vi "Main.vi"() -> ()   [LabVIEW 2021]
uses:
  <vilib>/gmath/NumericalOptimization/stopping criteria.ctl
  <vilib>/Platform/TimedLoop/XDataNode/timing_clust.ctl
  <vilib>/Platform/TimedLoop/XDataNode/nitl_modes.ctl
  <vilib>/Platform/TimedLoop/XDataNode/wakeup.ctl
  <vilib>/DAQmx/write.llb/DAQmx Write (Digital 1D Bool 1Chan 1Samp).vi
  <vilib>/DAQmx/write.llb/DAQmx Write (Analog 1D DBL NChan 1Samp).vi
  <vilib>/DAQmx/create/channels.llb/DAQmx Create Channel (DO-Digital Output).vi
  <vilib>/DAQmx/create/channels.llb/DAQmx Create Channel (AO-Voltage-Basic).vi
  <vilib>/DAQmx/create/channels.llb/DAQmx Create Channel (AI-Voltage-Basic).vi
  <vilib>/DAQmx/configure/timing.llb/DAQmx Timing (Sample Clock).vi
  <vilib>/DAQmx/miscellaneous.llb/DAQmx Fill In Error Info.vi
  <vilib>/platform/TimedLoop/XDataNode/XDataNode.xnode
  <vilib>/Platform/TimedLoop/XDataNode/XDNodeRunTimeDep.lvlib
  <vilib>/Analysis/NI_AALBase.lvlib
  <vilib>/Analysis/baseanly.llb/Real Dot Product.vi
  <vilib>/gmath/NI_Gmath.lvlib
panel:
  in  "RBF 5":bool=TRUE
  in  "State x 3":cluster{"Number":i32, "x_0":dbl, "x_f":dbl}={"Number"=20, "x_0"=0.0, "x_f"=500.0}
  out "XY Graph 3":cluster{dbl[], dbl[]}[](graph)=[{[0.0, 26.31578947368421, 52.63157894736842, 78.94736842105263, 105.26315789473684, 131.57894736842104, 157.89473684210526, 184.21052631578945, 210.52631578947367, 236.8421052631579, 263.1578947368421, 289.4736842105263, 315.7894736842105, 342.10526315789474, 368.4210526315789, 394.7368421052631, 421.05263157894734, 447.36842105263156, 473.6842105263158, 499.99999999999994], [-1.87, -1.8414422208867078, -1.7583590718201578, -1.6281335147614857, -1.4618588659589593, -1.2727815045556152, -1.0745713204427367, -0.879730430835235, -0.6983883150844216, -0.5376223240442685, -0.40131981493157487, -0.2904938166741144, -0.20389950050143207, -0.13878048824938563, -0.09159539506910583, -0.058620814615532306, -0.03638002877625406, -0.02189309729851222, -0.012775689731560116, -0.007229270660814157]}, {[0.0, 26.31578947368421, 52.63157894736842, 78.94736842105263, 105.26315789473684, 131.57894736842104, 157.89473684210526, 184.21052631578945, 210.52631578947367, 236.8421052631579, 263.1578947368421, 289.4736842105263, 315.7894736842105, 342.10526315789474, 368.4210526315789, 394.7368421052631, 421.05263157894734, 447.36842105263156, 473.6842105263158, 499.99999999999994], [-0.5809906464511002, -0.7664296918795039, -0.9804116917090333, -1.2161233359855126, -1.462782454638376, -1.706140698730468, -1.9296694582665639, -2.116332899482121, -2.2507021378374863, -2.3210529255377237, -2.3210529255377237, -2.2507021378374863, -2.1163328994821216, -1.9296694582665639, -1.7061406987304686, -1.4627824546383765, -1.2161233359855128, -0.9804116917090334, -0.7664296918795039, -0.5809906464511005]}, {[0.0, 26.31578947368421, 52.63157894736842, 78.94736842105263, 105.26315789473684, 131.57894736842104, 157.89473684210526, 184.21052631578945, 210.52631578947367, 236.8421052631579, 263.1578947368421, 289.4736842105263, 315.7894736842105, 342.10526315789474, 368.4210526315789, 394.7368421052631, 421.05263157894734, 447.36842105263156, 473.6842105263158, 499.99999999999994], [0.006649382639893229, 0.011750901785178288, 0.020136966499166315, 0.03346184464981654, 0.05391861023460723, 0.08424817086570154, 0.12764836352349906, 0.18754392559490007, 0.2671921736253885, 0.3691283859263683, 0.49449753869312374, 0.6423678620027834, 0.8091638187361518, 0.9883757599794155, 1.1706867314629184, 1.3445974595986148, 1.4975345697271418, 1.6173142264869897, 1.6937329518316242, 1.72]}, {[0.0, 26.31578947368421, 52.63157894736842, 78.94736842105263, 105.26315789473684, 131.57894736842104, 157.89473684210526, 184.21052631578945, 210.52631578947367, 236.8421052631579, 263.1578947368421, 289.4736842105263, 315.7894736842105, 342.10526315789474, 368.4210526315789, 394.7368421052631, 421.05263157894734, 447.36842105263156, 473.6842105263158, 499.99999999999994], [-2.444341263811207, -2.5961210109810335, -2.7186337970300247, -2.8107950060971816, -2.8707227103627284, -2.8946740324203812, -2.8765924151858018, -2.808519404722456, -2.6818982792965196, -2.489546863655624, -2.2278752017761745, -1.898828092508817, -1.5110685812474018, -1.080074186536534, -0.627049362336656, -0.17680580965529402, 0.2450312049653749, 0.6150094374794441, 0.9145275702205602, 1.1317800828880853]}]
  in  "RBF 4":cluster{"STD":dbl, "Number":i32}={"STD"=150.0, "Number"=3}
  out "RBF Output 3":dbl(slide)=-2.8000715957430593 scale=-40.0..50.0
  out "Weights 3":dbl[](array[slide])=[-1.87, -2.33, 1.72] scale=0.0..100.0
  out "100ms Finished Late?":bool
  out "100ms":i64=2
  out "1ms Finished Late?":bool
  in  "Encoder":bool
  in  "Tension Control Gains":T1(array[cluster])=[{"proportional gain (Kc)"=0.03, "integral time (Ti, min)"=0.0, "derivative time (Td, min)"=0.0}, {"proportional gain (Kc)"=0.03, "integral time (Ti, min)"=0.0, "derivative time (Td, min)"=0.0}, {"proportional gain (Kc)"=0.03, "integral time (Ti, min)"=0.0, "derivative time (Td, min)"=0.0}] {"derivative time (Td, min)" format="%.3f"; "integral time (Ti, min)" format="%.3f"; "proportional gain (Kc)" format="%.3f"}
  out "Ref Position (mm)":dbl
  out "1ms":i64=2
  in  "stop":bool
  out "10ms Finished Late?":bool
  out "10ms":i64=2
  in  "QP Stopping Criteria":T2={"function tolerance"=0.001, "parameter tolerance"=1e-05, "max iterations"=50, "max function calls"=50, "gradient tolerance"=1e-05, "max time (sec)"=0.01}
  in  "QP?":bool
  out "QP Solved":bool
  in  "Record?":bool
  in  "Trajectory":i32(knob) scale=0.0..2.0
  # "CONTROL"
  # "DEVEL"
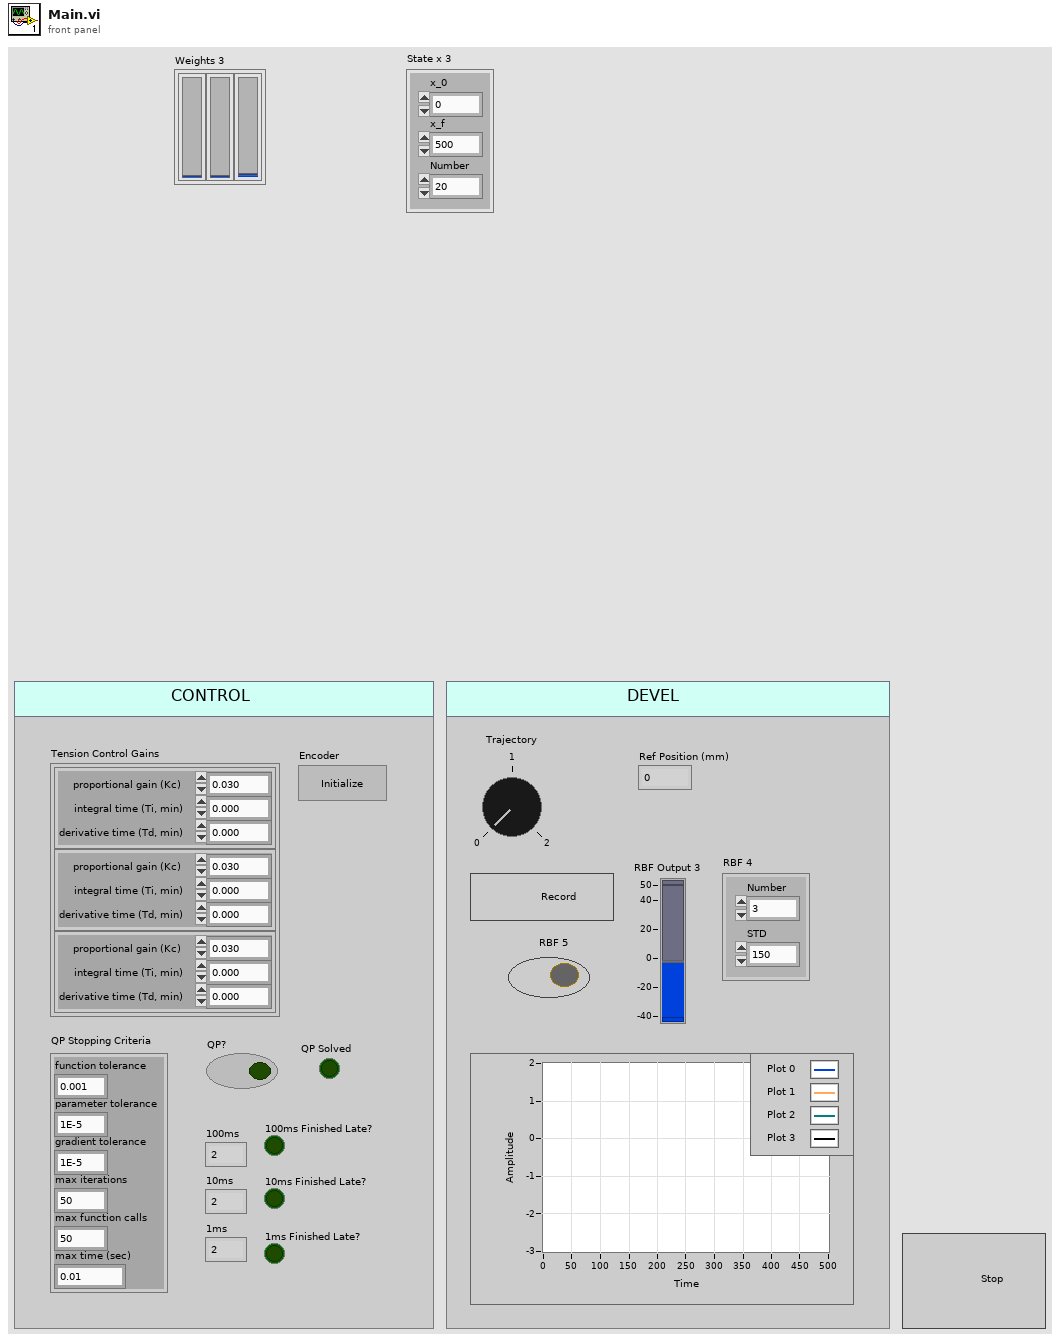
[diagram p1: front panel]
types:
  T1 = cluster{"proportional gain (Kc)":dbl, "integral time (Ti, min)":dbl, "derivative time (Td, min)":dbl}[]
  T2 = typedef "NI_Gmath.lvlib/stopping criteria.ctl" = cluster{"function tolerance":dbl, "parameter tolerance":dbl, "max iterations":i32, "max function calls":i32, "gradient tolerance":dbl, "max time (sec)":dbl}
  T3 = typedef "XDNodeRunTimeDep.lvlib/timing_clust.ctl" = cluster{"Expected End [f-1]":u64, "Actual End [f-1]":u64, "Finished Late? [f-1]":bool, "Expected End [i-1]":u64, "Actual End [i-1]":u64, "Finished Late? [i-1]":bool, "Expected Start [i]":u64, "Actual Start [i]":u64, "Expected Start [f]":u64, "Actual Start [f]":u64, "Source Name":string, "Structure Name":string, "Period":i64, "Deadline":i64, "Offset":i64, "Start":i64, "Priority":i32, "Timeout":i32, "Mode":T4, "Wakeup Reason":T5, "Error":errorcluster, "Source Type":string, "Secondary Source Type":string, "Global End Time":u64, "Global Start Time":u64, "Frame Duration":u64, "Iteration Duration":u64, "Assigned CPU":i32, "I/O Scan Engine Mode":u32}
  T4 = typedef "XDNodeRunTimeDep.lvlib/nitl_modes.ctl" = enum32{"No Change", "Process missed periods, maintain original phase", "Discard missed periods, maintain original phase", "Process missed periods, ignore original phase", "Discard missed periods, ignore original phase"}
  T5 = typedef "XDNodeRunTimeDep.lvlib/wakeup.ctl" = enum32{"Normal", "Aborted", "Asynchronous wakeup", "Timing source error", "Timed loop error", "Timeout"}
  T6 = typedef "NI_Matrix.lvlib/RealMatrix.ctl" = dbl[][]
  T7 = enum16{"open", "open or create", "create or replace", "create", "open (read-only)"}
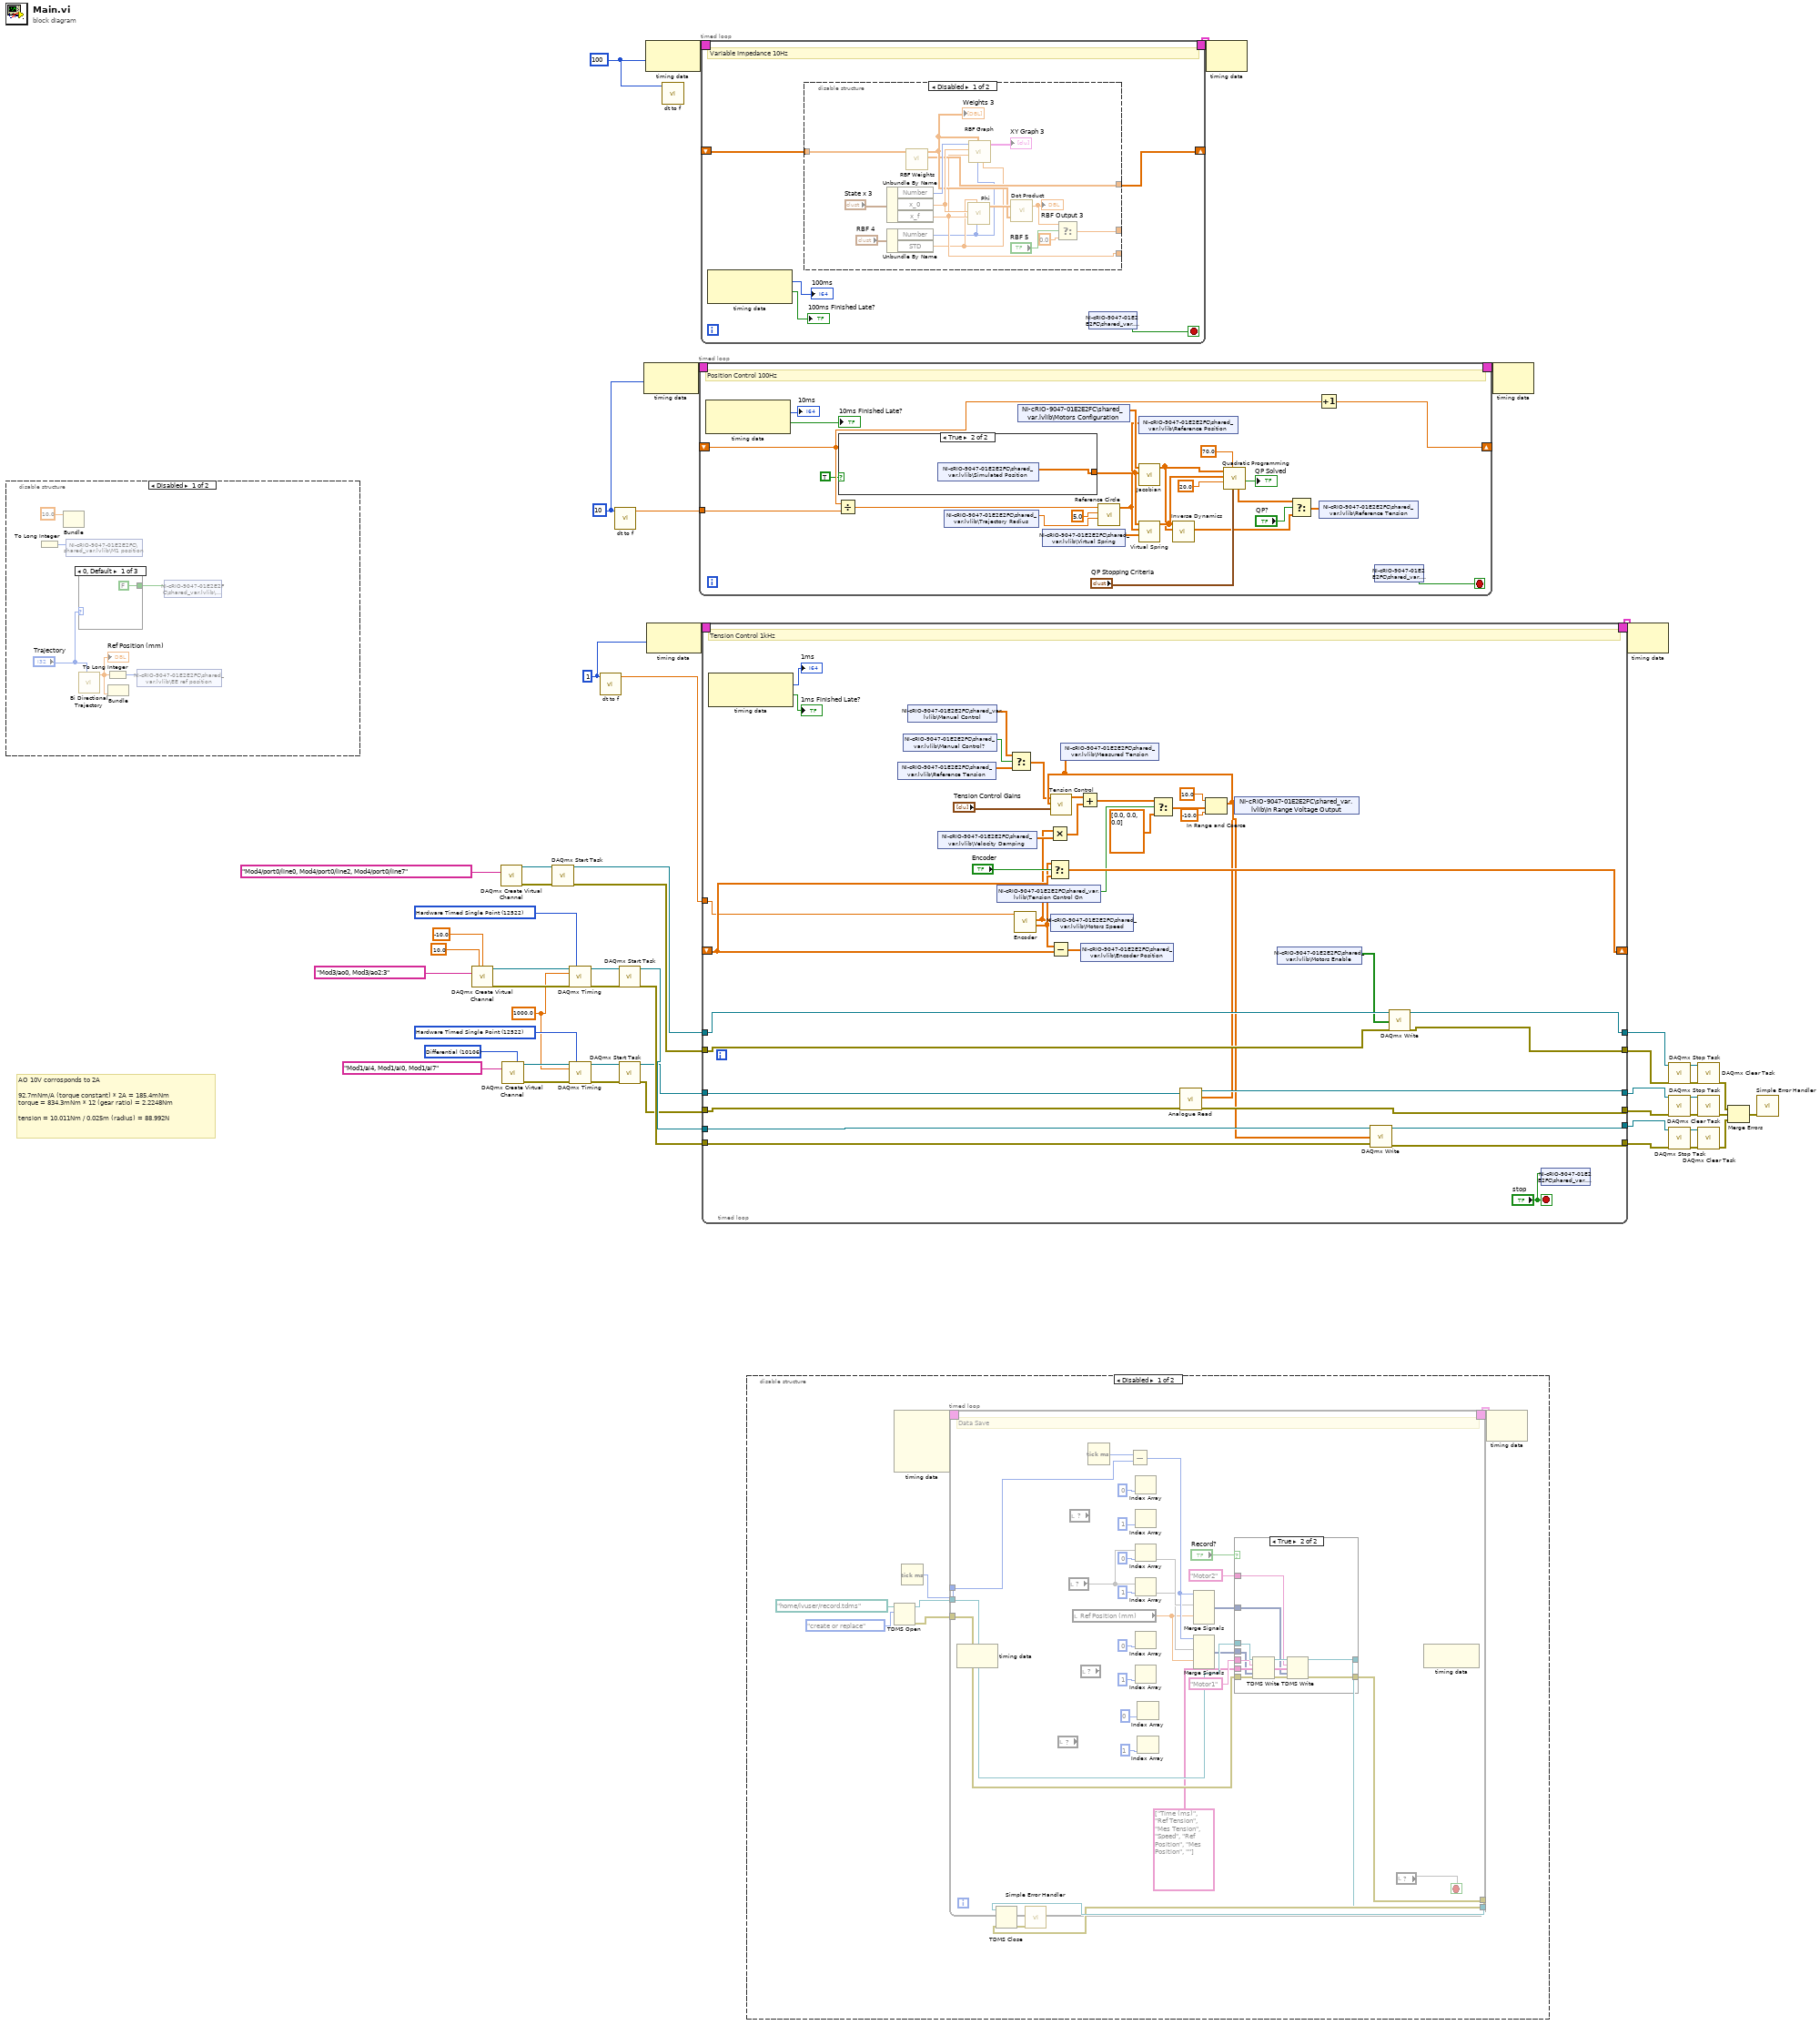
[diagram p0: block diagram]
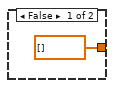
[diagram p3: hidden frame]
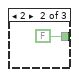
[diagram p4: hidden frame]
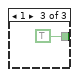
[diagram p5: hidden frame]
diagram:
  w1 = i64 100 ("Period 3")
  w5 = i64 10 ("Period 3")
  w14 = 12522 items=["Finite Samples"=10178, "Continuous Samples"=10123, "Hardware Timed Single Point"=12522] ("sample mode")
  w16 = 12522 items=["Finite Samples"=10178, "Continuous Samples"=10123, "Hardware Timed Single Point"=12522] ("sample mode")
  w8 = 1000.0 ("rate")
  w21 = i64 1 ("Period")
  w24 = 10106 items=["Default"=-1, "RSE"=10083, "NRSE"=10078, "Differential"=10106, "Pseudodifferential"=12529] ("input terminal configuration")
  # "AO 10V corrosponds to 2A\n\n92.7mNm/A (torque constant) * 2A = 185.4mNm\ntorque = 834.3mNm * 12 (gear ratio) = 2.2248Nm\n\ntension = 10.011Nm / 0.025m (radius) = 88.992N"
  n1 = disable-structure shown="Disabled" {
    frame Disabled {
      n2 = To Long Integer() -> (32bit integer=w57:i32)  [unwired: 1 in]
      n3 = Bundle("y"=10.0) -> ()  [unwired: 3 in, 1 out]
      n4 = shared-variable "NI-cRIO-9047-01E2E2FC\\shared_var.lvlib\\M1 position"(w57) -> ()  [unwired: 1 in, 1 out]
      n5 = case shown="0, Default" "Trajectory" {
        tunnel: [FALSE FALSE TRUE] -> w54
        frame 0, Default {
        }
        frame 2 {
        }
        frame 1 {
        }
      }
      n6 = call "Bi Directional Trajectory.vi"("Traj Start"="Trajectory") -> ("Output (mm)"=w56:dbl)  [unwired: 8 in, 2 out]
      "Ref Position (mm)" <- w56
      n7 = To Long Integer(number=w56) -> (32bit integer=w58:i32)
      n8 = Bundle("Output (mm)"=w56) -> ()  [unwired: 2 in, 1 out]
      n9 = shared-variable "NI-cRIO-9047-01E2E2FC\\shared_var.lvlib\\EE ref position"(w58) -> ()  [unwired: 1 in, 1 out]
      n10 = shared-variable "NI-cRIO-9047-01E2E2FC\\shared_var.lvlib\\Trigger"(w54) -> ()  [unwired: 1 in, 1 out]
    }
    frame Enabled {
    }
  }
  n11 = call-poly <vilib>:"DAQmx Create Virtual Channel.vi"("maximum value"=10.0 ("AO max"), "minimum value"=-10.0 ("AO min"), "physical channels"=tag "Mod3/ao0, Mod3/ao2:3" ("Physical Channel(s)")) -> ("task out"=w13:refnum<k21>, "error out"=w11:errorcluster)  [unwired: 11 in]
  n12 = call-poly <vilib>:"DAQmx Create Virtual Channel.vi"("lines"=tag "Mod4/port0/line0, Mod4/port0/line2, Mod4/port0/line7") -> ("task out"=w15:refnum<k21>, "error out"=w46:errorcluster)  [unwired: 13 in]
  n13 = call-poly <vilib>:"DAQmx Create Virtual Channel.vi"("input terminal configuration"=w24, "physical channels"=tag "Mod1/ai4, Mod1/ai0, Mod1/ai7") -> ("task out"=w20:refnum<k21>, "error out"=w19:errorcluster)  [unwired: 12 in]
  n14 = call <vilib>:"DAQmx Start Task.vi"("task/channels in"=w15, "error in"=w46) -> ("task out"=w44:refnum<k21>, "error out"=w43:errorcluster)  [unwired: 12 in]
  n15 = call-poly <vilib>:"DAQmx Timing.vi"("task/channels in"=w13, "sample mode"=w14, "rate"=w8, "error in"=w11) -> ("task out"=w12:refnum<k21>, "error out"=w10:errorcluster)  [unwired: 10 in]
  n16 = call-poly <vilib>:"DAQmx Timing.vi"("task/channels in"=w20, "sample mode"=w16, "rate"=w8, "error in"=w19) -> ("task out"=w17:refnum<k21>, "error out"=w18:errorcluster)  [unwired: 10 in]
  n17 = call "dt to f.vi"("Period"=w21) -> ("Frequency"=w9:dbl)  [unwired: 10 in]
  n18 = call "dt to f.vi"("Period"=w5) -> ("Frequency"=w4:dbl)  [unwired: 10 in]
  n19 = call <vilib>:"DAQmx Start Task.vi"("task/channels in"=w12, "error in"=w10) -> ("task out"=w48:refnum<k21>, "error out"=w47:errorcluster)  [unwired: 12 in]
  n20 = call <vilib>:"DAQmx Start Task.vi"("task/channels in"=w17, "error in"=w18) -> ("task out"=w37:refnum<k21>, "error out"=w36:errorcluster)  [unwired: 12 in]
  n21 = node-c288(w5) -> (w7:T3)
  n22 = node-c288(w1) -> (w3:T3)
  n23 = node-c288(w21) -> (w23:T3)
  n24 = call "dt to f.vi"("Period"=w1) -> ()  [unwired: 10 in, 1 out]
  n25 = timed-loop {
    timing: w7 -> [_]
    timing-out: [_] -> w6
    shift-right: [w83] -> _
    shift-left: _ -> [w82]
    tunnel: w4 -> [w62]
    stop <- w63 stop-if-true
    # "Position Control 100Hz"
    n26 = node-c288() -> (→"10ms":i64, →"10ms Finished Late?":bool)  [unwired: 1 in]
    n27 = Divide(x=w82, y=w62) -> (x/y=w72:dbl)
    n28 = case shown="True" TRUE {
      tunnel: [dbl[] [] w90] -> w71
      frame False {
      }
      frame True {
        n29 = shared-variable "NI-cRIO-9047-01E2E2FC\\shared_var.lvlib\\Simulated Position"() -> (w90:dbl[])  [unwired: 1 in, 1 out]
      }
    }
    n30 = shared-variable "NI-cRIO-9047-01E2E2FC\\shared_var.lvlib\\Trajectory Radius"() -> (w73:dbl)  [unwired: 1 in, 1 out]
    n31 = shared-variable "NI-cRIO-9047-01E2E2FC\\shared_var.lvlib\\Motors Configuration"() -> (w75:dbl[][])  [unwired: 1 in, 1 out]
    n32 = shared-variable "NI-cRIO-9047-01E2E2FC\\shared_var.lvlib\\Virtual Spring"() -> (w79:dbl[])  [unwired: 1 in, 1 out]
    n33 = call "Reference Circle.vi"("Radius"=w73, "Frequency"=5.0 ("y"), "Time"=w72) -> ("Reference Position"=w67:dbl[])  [unwired: 8 in]
    n34 = shared-variable "NI-cRIO-9047-01E2E2FC\\shared_var.lvlib\\Reference Position"(w67) -> ()  [unwired: 1 in, 1 out]
    n35 = call "Jacobian.vi"("EE Position"=w71, "Motor Position"=w75) -> ("Jacobian"=w69:T6)  [unwired: 9 in]
    n36 = call "Virtual Spring.vi"("P Gain"=w79, "Reference Position"=w67, "Actual Position"=w71) -> ("Desired Force Matrix"=w77:T6)  [unwired: 8 in]
    n37 = call "Inverse Dynamics.vi"("Jacobian Matrix"=w69, "F desired Matrix"=w77) -> ("Reference Tension"=w76:dbl[])  [unwired: 9 in]
    n38 = call "Quadratic Programming.vi"("stopping Criteria"="QP Stopping Criteria", "UB"=70.0, "LB"=20.0, "Desired Force Matrix"=w77, "Jacobian"=w69) -> ("Boolean"=→"QP Solved":bool, "minimum"=w74:dbl[])  [unwired: 3 in, 2 out]
    n39 = Select(t=w74, s="QP?", f=w76) -> (s? t:f=w66:dbl[])
    n40 = Increment(x=w82) -> (x+1=w83:dbl)
    n41 = shared-variable "NI-cRIO-9047-01E2E2FC\\shared_var.lvlib\\Reference Tension"(w66) -> ()  [unwired: 1 in, 1 out]
    n42 = shared-variable "NI-cRIO-9047-01E2E2FC\\shared_var.lvlib\\Stop"() -> (w63:bool)  [unwired: 1 in, 1 out]
  }
  n43 = timed-loop {
    timing: w3 -> [_]
    timing-out: [_] -> w2
    shift-right: [w95] -> _
    shift-left: _ -> [w96]
    stop <- w92 stop-if-true
    # "Variable Impedance 10Hz"
    n44 = node-c288() -> (→"100ms":i64, →"100ms Finished Late?":bool)  [unwired: 1 in]
    n45 = disable-structure shown="Disabled" {
      disable-tunnel: w96 -> [w106 _]
      disable-tunnel: [w105 _] -> w95
      disable-tunnel: [w103 _] -> _
      disable-tunnel: [w100 _] -> _
      frame Disabled {
        n46 = Unbundle By Name("State x 3") -> ("Number"=w112:i32, "x_0"=w109:dbl, "x_f"=w103:dbl)
        n47 = Unbundle By Name("RBF 4") -> ("Number"=w101:i32, "STD"=w102:dbl)
        n48 = call "RBF Weights.vi"("Array of Double in"=w106) -> ("Array of Double out"=w105:dbl[], "Array of Double 3"=w107:dbl[])  [unwired: 9 in]
        "Weights 3" <- w107
        n49 = call "Phi.vi"("Number"=w101, "STD"=w102, "x_f"=w103, "x_0"=w109) -> ("Array"=w108:dbl[])  [unwired: 7 in]
        n50 = call "RBF Graph.vi"("STD"=w102, "Number"=w101, "Array of Double 3"=w107, "x_f"=w103, "x_0"=w109, "Number 2"=w112) -> ("Array"=→"XY Graph 3":cluster{dbl[], dbl[]}[])  [unwired: 5 in]
        n51 = call-poly <vilib>:"Dot Product.vi"("Y Vector"=w107, "X Vector"=w108) -> ("X * Y"=w104:dbl)  [unwired: 1 out]
        "RBF Output 3" <- w104
        n52 = Select(t=w104, s="RBF 5", f=0.0) -> (s? t:f=w100:dbl)
      }
      frame Enabled {
      }
    }
    n53 = shared-variable "NI-cRIO-9047-01E2E2FC\\shared_var.lvlib\\Stop"() -> (w92:bool)  [unwired: 1 in, 1 out]
  }
  n54 = timed-loop {
    tunnel: [w155] -> w52
    tunnel: [w154] -> w51
    tunnel: [w143] -> w50
    tunnel: [w146] -> w49
    tunnel: w37 -> [w152]
    tunnel: w36 -> [w151]
    tunnel: w48 -> [w142]
    tunnel: w47 -> [w153]
    tunnel: w44 -> [w150]
    tunnel: w43 -> [w149]
    tunnel: [w148] -> w40
    tunnel: [w147] -> w39
    shift-right: [w145] -> _
    shift-left: _ -> [w144]
    timing: w23 -> [_]
    timing-out: [_] -> w22
    tunnel: w9 -> [w123]
    stop <- "stop" stop-if-true
    # "Tension Control 1kHz"
    n55 = node-c288() -> (→"1ms":i64, →"1ms Finished Late?":bool)  [unwired: 1 in]
    n56 = shared-variable "NI-cRIO-9047-01E2E2FC\\shared_var.lvlib\\Reference Tension"() -> (w118:dbl[])  [unwired: 1 in, 1 out]
    n57 = shared-variable "NI-cRIO-9047-01E2E2FC\\shared_var.lvlib\\Manual Control?"() -> (w120:bool)  [unwired: 1 in, 1 out]
    n58 = shared-variable "NI-cRIO-9047-01E2E2FC\\shared_var.lvlib\\Manual Control"() -> (w119:dbl[])  [unwired: 1 in, 1 out]
    n59 = shared-variable "NI-cRIO-9047-01E2E2FC\\shared_var.lvlib\\Velocity Damping"() -> (w132:dbl[])  [unwired: 1 in, 1 out]
    n60 = shared-variable "NI-cRIO-9047-01E2E2FC\\shared_var.lvlib\\Tension Control On"() -> (w125:bool)  [unwired: 1 in, 1 out]
    n61 = Select(t=w119, s=w120, f=w118) -> (s? t:f=w121:dbl[])
    n62 = call "Encoder.vi"("Frequency"=w123) -> ("Encoder Position (mm)"=w129:dbl[], "RPM"=w124:dbl[])  [unwired: 9 in]
    n63 = Multiply(x=w124, y=w132) -> (x*y=w127:dbl[])
    n64 = Select(t=w129, s="Encoder", f=w144) -> (s? t:f=w145:dbl[])
    n65 = Subtract(x=w129, y=w144) -> (x-y=w128:dbl[])
    n66 = shared-variable "NI-cRIO-9047-01E2E2FC\\shared_var.lvlib\\Motors Speed"(w124) -> ()  [unwired: 1 in, 1 out]
    n67 = shared-variable "NI-cRIO-9047-01E2E2FC\\shared_var.lvlib\\Encoder Position"(w128) -> ()  [unwired: 1 in, 1 out]
    n68 = call "Analogue Read.vi"("error in"=w151, "task/channels in"=w152) -> ("error out"=w146:errorcluster, "Measured Tension"=w122:dbl[], "task out"=w143:refnum<k21>)  [unwired: 7 in]
    n69 = call "Tension Control.vi"("PID gains"="Tension Control Gains", "Measured Tension"=w122, "Reference Tension"=w121) -> ("Voltage Output"=w131:dbl[])  [unwired: 8 in]
    n70 = shared-variable "NI-cRIO-9047-01E2E2FC\\shared_var.lvlib\\Measured Tension"(w122) -> ()  [unwired: 1 in, 1 out]
    n71 = Add(x=w131, y=w127) -> (x+y=w130:dbl[])
    n72 = Select(t=w130, s=w125, f=dbl[] [0.0, 0.0, 0.0]) -> (s? t:f=w139:dbl[])
    n73 = In Range and Coerce(upper limit=10.0, x=w139, lower limit=-10.0) -> (coerced(x)=w135:dbl[])  [unwired: 1 out]
    n74 = shared-variable "NI-cRIO-9047-01E2E2FC\\shared_var.lvlib\\In Range Voltage Output"(w135) -> ()  [unwired: 1 in, 1 out]
    n75 = shared-variable "NI-cRIO-9047-01E2E2FC\\shared_var.lvlib\\Motors Enable"() -> (w136:bool[])  [unwired: 1 in, 1 out]
    n76 = call-poly <vilib>:"DAQmx Write.vi"("task/channels in"=w142, "data"=w135, "error in"=w153) -> ("task out"=w155:refnum<k21>, "error out"=w154:errorcluster)  [unwired: 10 in, 1 out]
    n77 = call-poly <vilib>:"DAQmx Write.vi"("task/channels in"=w150, "data"=w136, "error in"=w149) -> ("task out"=w148:refnum<k21>, "error out"=w147:errorcluster)  [unwired: 10 in, 1 out]
    n78 = shared-variable "NI-cRIO-9047-01E2E2FC\\shared_var.lvlib\\Stop"("stop") -> ()  [unwired: 1 in, 1 out]
  }
  n79 = disable-structure shown="Disabled" {
    frame Disabled {
      n80 = TDMS Open(10:T7."create or replace" ("operation (0:open)"), 11:path "/home/lvuser/record.tdms" ("file path")) -> (0:w163:errorcluster, 3:w167:refnum<k34>)  [unwired: 5 in]
      n81 = node-c288() -> (w169:T3)  [unwired: 4 in]
      n82 = Tick Count (ms)() -> (millisecond timer value=w160:u32)
      n83 = timed-loop {
        tunnel: w167 -> [w195]
        tunnel: [w184] -> w166
        tunnel: [w192] -> w164
        tunnel: w163 -> [w194]
        tunnel: w160 -> [w186]
        timing: w169 -> [_]
        timing-out: [_] -> w168
        stop <- w182 stop-if-true
        # "Data Save"
        n84 = node-c288() -> ()  [unwired: 1 in, 1 out]
        n85 = local read item#-1() -> ()  [unwired: 1 out]
        n86 = local read item#-1() -> (w179)
        n87 = local read item#-1() -> ()  [unwired: 1 out]
        n88 = local read "Ref Position (mm)"() -> (w172:dbl)
        n89 = local read item#-1() -> ()  [unwired: 1 out]
        n90 = Tick Count (ms)() -> (millisecond timer value=w187:u32)
        n91 = Subtract(x=w187, y=w186) -> (x-y=w185:u32)
        n92 = Index Array(index=0) -> ()  [unwired: 1 in, 1 out]
        n93 = Index Array(index=1) -> ()  [unwired: 1 in, 1 out]
        n94 = Index Array(array=w179, index=0) -> (element=w178)
        n95 = Index Array(array=w179, index=1) -> (element=w177)
        n96 = Index Array(index=0) -> ()  [unwired: 1 in, 1 out]
        n97 = Index Array(index=1) -> ()  [unwired: 1 in, 1 out]
        n98 = Index Array(index=0) -> ()  [unwired: 1 in, 1 out]
        n99 = Index Array(index=1) -> ()  [unwired: 1 in, 1 out]
        n100 = Merge Signals(w185, w178, w172) -> (w188:dynamicdata)  [unwired: 3 in]
        n101 = Merge Signals(w185, w177, w172) -> (w189:dynamicdata)  [unwired: 3 in]
        n102 = case shown="True" "Record?" {
          tunnel: w195 -> [w196 w209]
          tunnel: w194 -> [w197 w208]
          tunnel: "Motor1" ("group name in (Untitled)") -> [_ w207]
          tunnel: [w197 w205] -> w192
          tunnel: [w196 w203] -> w184
          tunnel: "Motor2" ("group name in (Untitled)") -> [_ w202]
          tunnel: string[] ["Time (ms)", "Ref Tension", "Mes Tension", "Speed", "Ref Position", "Mes Position", ""] ("channel name(s) in (Untitled)") -> [_ w201]
          tunnel: w189 -> [_ w199]
          tunnel: w188 -> [_ w198]
          frame False {
          }
          frame True {
            n103 = TDMS Write(0:w209, 5:w207, 7:w201, 9:w199, 11:w208) -> (4:w204:refnum<k34>, 8:w200:string[], 15:w206:errorcluster)  [unwired: 1 in, 1 out]
            n104 = TDMS Write(0:w204, 5:w202, 7:w200, 9:w198, 11:w206) -> (4:w203:refnum<k34>, 15:w205:errorcluster)  [unwired: 1 in, 2 out]
          }
        }
        n105 = local read item#-1() -> (w182)
        n106 = node-c288() -> ()  [unwired: 1 in, 1 out]
      }
      n107 = TDMS Close(8:w164, 11:w166) -> (0:w165:errorcluster)  [unwired: 1 out]
      n108 = call <vilib>:"Simple Error Handler.vi"("error in (no error)"=w165) -> ()  [unwired: 4 in, 5 out]
      n109 = node-c288(w168) -> ()  [unwired: 1 out]
    }
    frame Enabled {
    }
  }
  n110 = node-c288(w2) -> ()  [unwired: 1 out]
  n111 = node-c288(w6) -> ()  [unwired: 1 out]
  n112 = node-c288(w22) -> ()  [unwired: 1 out]
  n113 = call <vilib>:"DAQmx Stop Task.vi"("task/channels in"=w40, "error in"=w39) -> ("task out"=w42:refnum<k21>, "error out"=w41:errorcluster)  [unwired: 12 in]
  n114 = call <vilib>:"DAQmx Stop Task.vi"("task/channels in"=w50, "error in"=w49) -> ("task out"=w30:refnum<k21>, "error out"=w29:errorcluster)  [unwired: 12 in]
  n115 = call <vilib>:"DAQmx Stop Task.vi"("task/channels in"=w52, "error in"=w51) -> ("task out"=w32:refnum<k21>, "error out"=w31:errorcluster)  [unwired: 12 in]
  n116 = call <vilib>:"DAQmx Clear Task.vi"("task in"=w42, "error in"=w41) -> ("error out"=w25:errorcluster)  [unwired: 13 in]
  n117 = call <vilib>:"DAQmx Clear Task.vi"("task in"=w30, "error in"=w29) -> ("error out"=w26:errorcluster)  [unwired: 13 in]
  n118 = call <vilib>:"DAQmx Clear Task.vi"("task in"=w32, "error in"=w31) -> ("error out"=w27:errorcluster)  [unwired: 13 in]
  n119 = Merge Errors(w25, w26, w27) -> (w28:errorcluster)
  n120 = call <vilib>:"Simple Error Handler.vi"("error in (no error)"=w28) -> ()  [unwired: 4 in, 5 out]
